vi "draw_overlay_3D.vi"(8 "error in (no error)":errorcluster, 10 "ImageCollection in":refnum<class "ImageCollection.lvclass">, 11 "GenericTrajectory in":refnum<class "TrajectoryDL091126GenericVoxel.lvclass">) -> (0 "error out":errorcluster, 2 "ImageCollection out":refnum<class "ImageCollection.lvclass">, 3 "GenericTrajectory out":refnum<class "TrajectoryDL091126GenericVoxel.lvclass">)   [LabVIEW 2010, in "TrajectoryDL091126GenericVoxel.lvclass"]
uses:
  TrajectoryDL091126GenericVoxel.lvclass
  common/classes/ImageCollection/ImageCollection/ImageCollection.lvclass
  common/classes/Image/Image/origin_type_enum.ctl
  common/classes/ErrorController/ErrorController/class_data.vi
  common/classes/Image/Image/Image.lvclass
  common/classes/SpaceVector/SpaceVector/SpaceVector.lvclass
  common/classes/ErrorController/ErrorController/ErrorController.lvclass
panel:
  in  "colour":u32(colorbox)=16711680
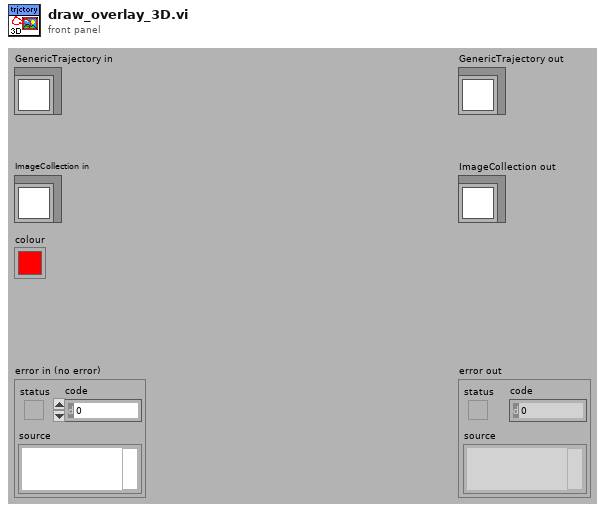
[diagram p1: front panel]
types:
  T1 = typedef "origin_type_enum.ctl" = enum16{"IMAQ origin", "middle of image"}
  T2 = typedef "TrajectoryDL091126GenericVoxel.lvclass/segment_cluster.ctl" = cluster{"x":dbl[unit][], "y":dbl[unit][], "z":dbl[unit][]}
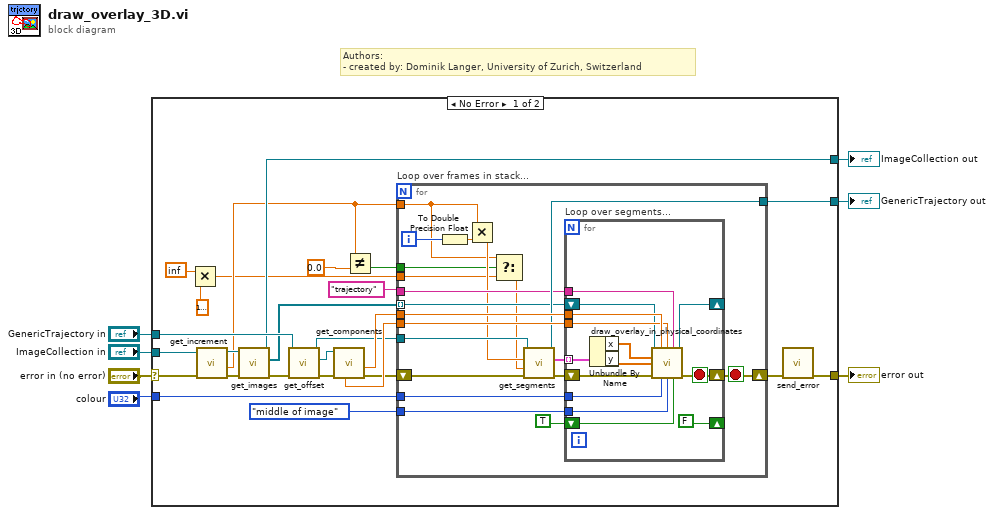
[diagram p0: block diagram]
diagram:
  # "Authors: \n- created by: Dominik Langer, University of Zurich, Switzerland"
  n1 = case shown="No Error" "error in (no error)" {
    selector: "error in (no error)" -> [w33 w70]
    tunnel: [w25 w70] -> w6
    tunnel: [w28 w69] -> w4
    tunnel: "GenericTrajectory in" -> [w29 w69]
    tunnel: "ImageCollection in" -> [w32 w68]
    tunnel: "colour" -> [w27 _]
    tunnel: [w26 w68] -> w1
    frame No Error {
      n2 = Multiply(x=inf, y=dbl[unit] 1e-06) -> (x*y=w8:dbl[unit])
      n3 = call "get_increment.vi"("error in (no error)"=w33, "ImageCollection in"=w32) -> ("error out"=w31:errorcluster, "z increment"=w10:dbl[unit], "ImageCollection out"=w30:refnum<class "ImageCollection.lvclass">)  [unwired: 5 in, 2 out]
      n4 = call-dynamic "get_images.vi"("error in (no error)"=w31, "ImageCollection.lvclass in"=w30) -> ("error out"=w18:errorcluster, "images"=w17:refnum<class "Image.lvclass">[], "ImageCollection.lvclass out"=w26:refnum<class "ImageCollection.lvclass">)  [unwired: 7 in]
      n5 = call "get_offset.vi"("error in (no error)"=w18, "GenericTrajectory.lvclass in"=w29) -> ("error out"=w23:errorcluster, "SpaceVector.lvclass"=w22:refnum<class "SpaceVector.lvclass">, "GenericTrajectory.lvclass out"=w14:refnum<class "TrajectoryDL091126GenericVoxel.lvclass">)  [unwired: 7 in]
      n6 = call "get_components.vi"("error in (no error)"=w23, "SpaceVector in"=w22) -> ("error out"=w15:errorcluster, "x"=w21:dbl[unit], "y"=w20:dbl[unit])  [unwired: 4 in, 3 out]
      n7 = Not Equal?(x=w10, y=dbl[unit] 0.0) -> (x != y?=w9:bool)
      n8 = for "Loop over frames in stack..." {
        tunnel: w14 -> [w42]
        tunnel: w21 -> [w53]
        tunnel: w20 -> [w52]
        tunnel: origin_type_enum."middle of image" ("origin") -> [w51]
        tunnel: w27 -> [w50]
        tunnel: w10 -> [w35]
        tunnel: [w46] -> w28
        tunnel: w17 -> [w44] mode=indexing
        tunnel: "trajectory" ("overlay group") -> [w43]
        tunnel: w9 -> [w38]
        tunnel: w8 -> [w37]
        shift-right: [w39] -> w24
        shift-left: w15 -> [w48]
        i -> [w45]
        stop <- w39 stop-if-true
        n9 = To Double Precision Float(number=w45) -> (double precision float=w49:dbl)
        n10 = Multiply(x=w35, y=w49) -> (x*y=w41:dbl[unit])
        n11 = Select(t=w35, s=w38, f=w37) -> (s? t:f=w36:dbl[unit])
        n12 = call-dynamic "get_segments.vi"("error in (no error)"=w48, "range"=w36, "offset"=w41, "GenericTrajectory in"=w42) -> ("error out"=w47:errorcluster, "segments"=w34:T2[], "GenericTrajectory out"=w46:refnum<class "TrajectoryDL091126GenericVoxel.lvclass">)  [unwired: 5 in]
        n13 = for "Loop over segments..." {
          tunnel: w53 -> [w67]
          tunnel: w52 -> [w66]
          tunnel: w51 -> [w65]
          tunnel: w50 -> [w64]
          tunnel: w34 -> [w62] mode=indexing
          shift-right: [w58] -> _
          shift-left: w44 -> [w59]
          tunnel: w43 -> [w57]
          shift-right: [FALSE] -> _
          shift-left: TRUE -> [w56]
          shift-right: [w54] -> w39
          shift-left: w47 -> [w63]
          stop <- w54 stop-if-true
          n14 = Unbundle By Name(w62) -> ("x"=w61:dbl[unit][], "y"=w60:dbl[unit][])
          n15 = call "draw_overlay_in_physical_coordinates.vi"("Image in"=w59, "x offset"=w67, "y offset"=w66, "overlay group"=w57, "x coordinates"=w61, "y coordinates"=w60, "error in (no error)"=w63, "colour"=w64, "origin"=w65, "clear previous overlay of this group?"=w56) -> ("Image out"=w58:refnum<class "Image.lvclass">, "error out"=w54:errorcluster)  [unwired: 4 in]
        }
      }
      n16 = call "send_error.vi"("error in (no error)"=w24) -> ("error out"=w25:errorcluster)  [unwired: 10 in]
    }
    frame Error {
    }
  }
  "error out" <- w6
  "GenericTrajectory out" <- w4
  "ImageCollection out" <- w1
